vi "Reference.vi"(8 "error in (no error)":errorcluster, 10 "Instrument":refnum<class "Instrument.lvclass">, 11 "InstrPtr in":refnum<class "InstrPtr.lvclass">) -> (0 "error out":errorcluster, 3 "InstrPtr out":refnum<class "InstrPtr.lvclass">)   [LabVIEW 2009, in "InstrPtr.lvclass"]
uses:
  InstrPtr.lvclass
  Instrument/Instrument.lvclass
  InstrPtr.lvclass/InstrPtr.ctl
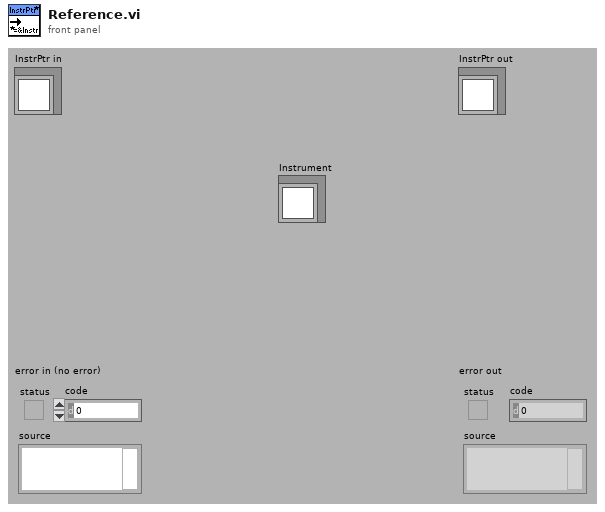
[diagram p1: front panel]
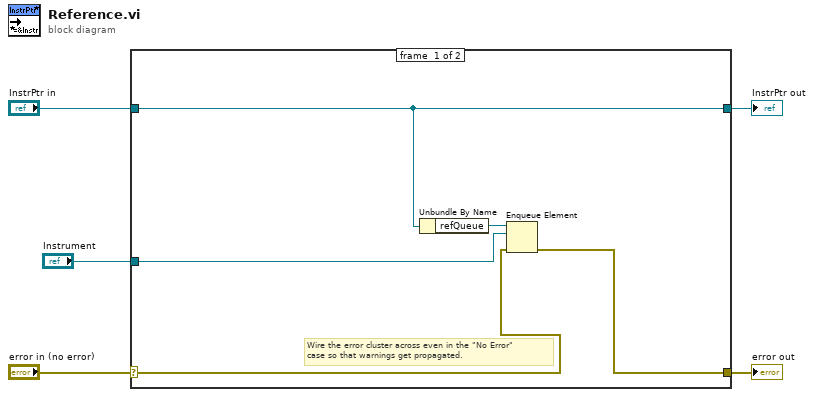
[diagram p0: block diagram]
diagram:
  n1 = case shown="No Error" "error in (no error)" {
    selector: "error in (no error)" -> [w8 w12]
    tunnel: [w7 w12] -> w4
    tunnel: [w9 w11] -> w2
    tunnel: "InstrPtr in" -> [w9 w11]
    tunnel: "Instrument" -> [w6 _]
    frame #0 {
      # "Wire the error cluster across even in the \"No Error\"\ncase so that warnings get propagated."
      n2 = Unbundle By Name(w9) -> ("refQueue"=w10:refnum<queue>)
      n3 = Enqueue Element(queue=w10, element=w6, error in (no error)=w8) -> (error out=w7:errorcluster)  [unwired: 3 out]
    }
    frame #1 {
    }
  }
  "error out" <- w4
  "InstrPtr out" <- w2
